vi "send_BrakeChecked.vi"(4 "Counter":i32, 5 "200/freq":i32=4, 6 "Active":bool, 7 "CAN ID":u32=561 format="%x", 8 "Message":T1 {"p Front" scale=0.0..100.0; "p Rear" scale=0.0..100.0}, 11 "CAN frame":T2[](array[typedef]) {"Data" format="%.0x"; "ArbitrationId" format="%.0x"; "Timestamp" format="%<%I:%M:%S%3u %p\n%m/%d/%Y>T"}) -> (3 "CAN frame out":T2[](array[typedef]) {"Data" format="%.0x"; "ArbitrationId" format="%.0x"; "Timestamp" format="%<%I:%M:%S%3u %p\n%m/%d/%Y>T"})   [LabVIEW 2017]
uses:
  <vilib>/nican/nican.llb/CanFrameTimed.ctl
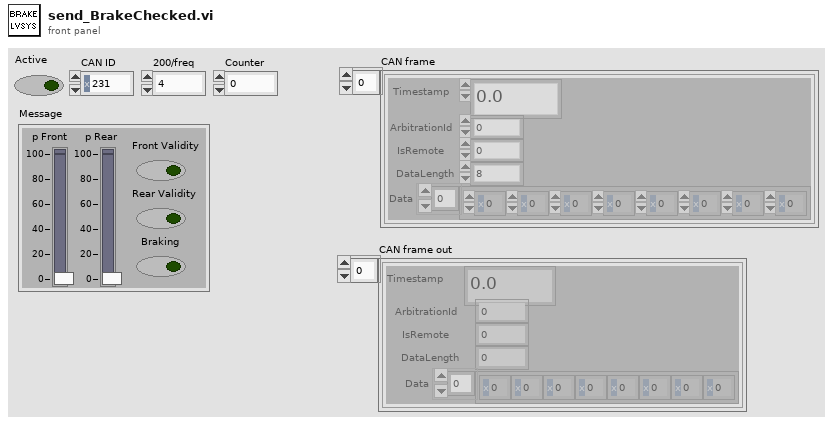
[diagram p1: front panel]
types:
  T1 = cluster{"Rear Validity":bool, "Front Validity":bool, "p Rear":dbl, "p Front":dbl, "Braking":bool}
  T2 = typedef "CanFrameTimed.ctl" = cluster{"Timestamp":dbl, "ArbitrationId":u32, "IsRemote":u8, "DataLength":u8, "Data":u8[]}
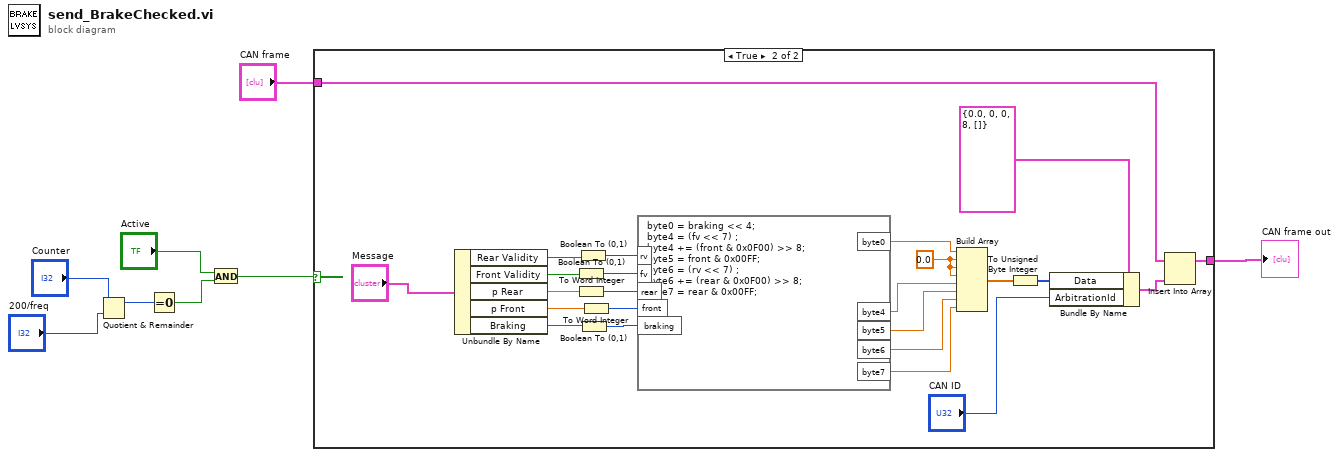
[diagram p0: block diagram]
diagram:
  n1 = Quotient & Remainder(x="Counter", y="200/freq") -> (x-y*floor(x/y)=w5:i32)  [unwired: 1 out]
  n2 = Equal To 0?(x=w5) -> (x = 0?=w3:bool)
  n3 = And(x="Active", y=w3) -> (x .and. y?=w2:bool)
  n4 = case shown="True" w2 {
    tunnel: "CAN frame" -> [w9 w30]
    tunnel: [w9 w28] -> w7
    frame False {
    }
    frame True {
      w10 = 0.0 ("element")
      n5 = Unbundle By Name("Message") -> ("Rear Validity"=w22:bool, "Front Validity"=w21:bool, "p Rear"=w19:dbl, "p Front"=w20:dbl, "Braking"=w18:bool)
      n6 = Boolean To (0,1)(Boolean=w21) -> (0, 1=w25:i16)
      n7 = To Word Integer(number=w19) -> (16bit integer=w26:i16)
      n8 = Boolean To (0,1)(Boolean=w22) -> (0, 1=w24:i16)
      n9 = Boolean To (0,1)(Boolean=w18) -> (0, 1=w17:i16)
      n10 = To Word Integer(number=w20) -> (16bit integer=w27:i16)
      n11 = formula code="byte0 = braking << 4;\nbyte4 = (fv << 7) ;\nbyte4 += (front & 0x0F00) >> 8;\nbyte5 = front & 0x00FF;\nbyte6 = (rv << 7) ;\nbyte6 += (rear & 0x0F00) >> 8;\nbyte7 = rear & 0x00FF;"("rear"=w26, "front"=w27, "rv"=w24, "fv"=w25, "braking"=w17) -> ("byte4"=w11:dbl, "byte5"=w12:dbl, "byte6"=w13:dbl, "byte7"=w14:dbl, "byte0"=w15:dbl)
      n12 = Build Array(w15, w10, w10, w10, w11, w12, w13, w14) -> (w33:dbl[])
      n13 = To Unsigned Byte Integer(number=w33) -> (unsigned 8bit integer=w32:u8[])
      n14 = Bundle By Name(cluster=T2 {"Timestamp"=0.0, "ArbitrationId"=0, "IsRemote"=0, "DataLength"=8, "Data"=[]} ("CAN frame"), "Data"=w32, "ArbitrationId"="CAN ID") -> (w29:T2)
      n15 = Insert Into Array(array=w30, new element=w29) -> (w28:T2[])  [unwired: 1 in]
    }
  }
  "CAN frame out" <- w7
